vi "MoveZmicroSwitch1_StepWiseMove.vi"(0 "Z":dbl=60.0, 1 "Zspeed":dbl=25.0, 2 "controller in":refnum<k24>, 3 "error in (no error)":errorcluster) -> (7 "MoveZ":string, 8 "controller out":refnum<k24>, 9 "data":bool[](array[boolean]), 10 "error out":errorcluster)   [LabVIEW 2019]
uses:
  C:/Users/TTUHEP/Documents/LabVIEW/Other Models/2010/Bin/Aerotech.A3200.dll
  Other Models/2010/Bin/Aerotech.A3200.dll
panel:
  # "Move along Z, abs coordinates, with speed v mm/s"
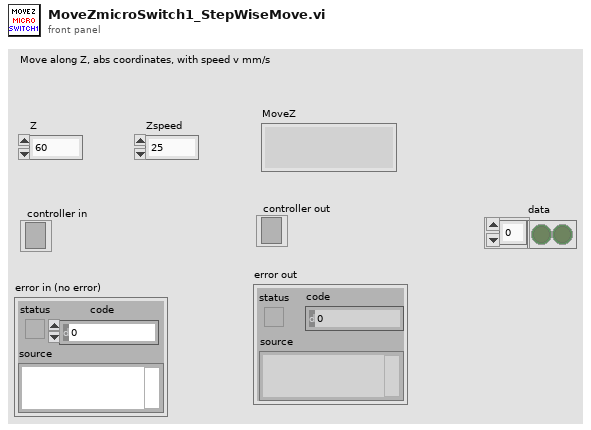
[diagram p1: front panel]
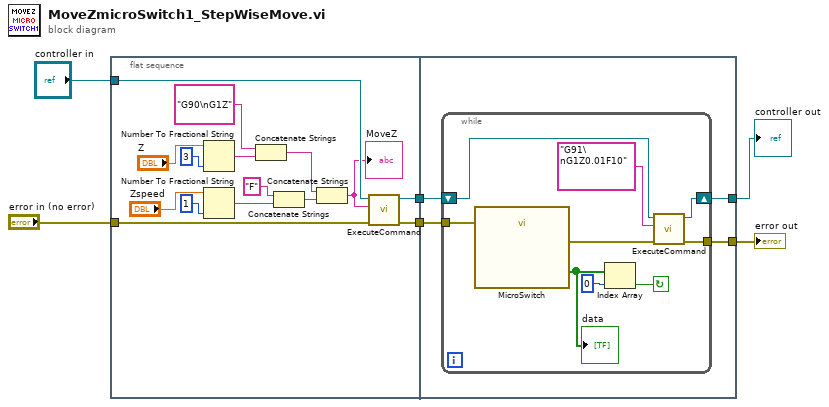
[diagram p0: block diagram]
diagram:
  n1 = flat-sequence {
    tunnel: "error in (no error)" -> [w21]
    tunnel: "controller in" -> [w20]
    tunnel: [w19] -> w6
    tunnel: [w18] -> w5
    tunnel: w6 -> [w24]
    tunnel: w5 -> [w25]
    tunnel: [w22] -> w1
    tunnel: [w23] -> w4
    frame #0 {
      n2 = Number To Fractional String(number="Z", precision (6)=i16 3) -> (F-format string=w13:string)  [unwired: 2 in]
      n3 = Number To Fractional String(number="Zspeed", precision (6)=i16 1) -> (F-format string=w16:string)  [unwired: 2 in]
      n4 = Concatenate Strings("G90\nG1Z", w13) -> (w14:string)
      n5 = Concatenate Strings("F" ("string"), w16) -> (w17:string)
      n6 = Concatenate Strings(w14, w17) -> (w7:string)
      "MoveZ" <- w7
      n7 = call "ExecuteCommand.vi"("error in (no error)"=w21, "Command Code"=w7, "controller in"=w20) -> ("error out"=w18:errorcluster, "controller out"=w19:refnum<k24>)  [unwired: 6 in, 1 out]
    }
    frame #1 {
      n8 = while {
        tunnel: [w26] -> w22
        tunnel: w25 -> [w34]
        shift-right: [w28] -> w23
        shift-left: w24 -> [w27]
        stop <- w32 continue-if-true
        n9 = call "MicroSwitch"("error in"=w34) -> ("data"=w33:bool[], "error out"=w29:errorcluster)  [unwired: 16 in, 1 out]
        "data" <- w33
        n10 = Index Array(array=w33, index=0) -> (element=w32:bool)
        n11 = call "ExecuteCommand.vi"("error in (no error)"=w29, "Command Code"="G91\nG1Z0.01F10", "controller in"=w27) -> ("error out"=w26:errorcluster, "controller out"=w28:refnum<k24>)  [unwired: 6 in, 1 out]
      }
    }
  }
  "controller out" <- w4
  "error out" <- w1
